vi "solar_qtimer Set (Message).vi"(8 "error in (no error)":errorcluster, 9 "DATA":variant, 10 "MSG":string, 11 "QTimer Name":string) -> (0 "error out":errorcluster)   [LabVIEW 2018]
doc: "[DEPRECIATED] This sets the message of the QTimer by name."
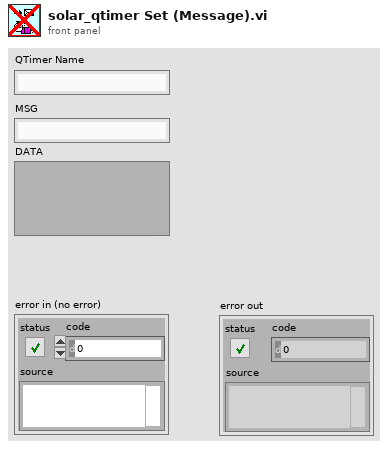
[diagram p1: front panel]
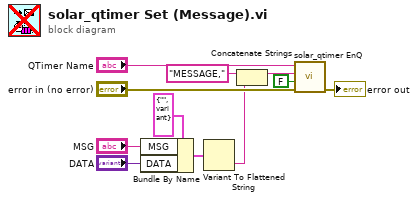
[diagram p0: block diagram]
diagram:
  n1 = Bundle By Name(cluster=cluster{"MSG":string, "DATA":variant} {"MSG"="", "DATA"=variant} ("Message"), "MSG"="MSG", "DATA"="DATA") -> (w4:cluster{"MSG":string, "DATA":variant})
  n2 = Variant To Flattened String(Variant=w4) -> (data string=w5:string)  [unwired: 1 out]
  n3 = Concatenate Strings("MESSAGE," ("CMD (\"\")"), w5) -> (w6:string)
  n4 = call "solar_qtimer EnQ.vi"("error in (no error)"="error in (no error)", "Create if not found? (F)"=FALSE, "CMD (\"\")"=w6, "QTimer Name"="QTimer Name") -> ("error out"=→"error out":errorcluster)  [unwired: 5 in, 2 out]
